vi "glb_static.vi"() -> ()   [LabVIEW 2014]
panel:
  in  "2-计算方法":string[](array[string])=["", "常数", "加", "减", "乘", "除", "微分", "积分", "幂运算", "散热量计算"]
  in  "2-变量来源_少运算":string[](array[string])=["", "测试模块1", "测试模块2", "测试模块3", "测试模块4", "测试模块5", "测试模块6", "测试模块7", "测试模块8", "cRIO", "GPS", "OBD", "冷却系统控制"]
  in  "2-变量来源_全部":string[](array[string])=["", "测试模块1", "测试模块2", "测试模块3", "测试模块4", "测试模块5", "测试模块6", "测试模块7", "测试模块8", "cRIO", "GPS", "OBD", "冷却系统控制", "运算"]
  in  "连接状态_OBD":bool
  in  "连接状态_GPS":bool
  in  "网络流2写入到的元素数量":i64
  in  "网络流2信息":T1={"cRIO名称"="RT", "读取方名称"="XpdGhnv3vatyoD3", "写入方名称 "="zGR2YhZf2vjoZ5U", "网络流大小"=10240, "网络流超时"=5000, "元素类型"={"消息"="", "数据"=variant}}
  in  "网络流2读取方端点":refnum<k21>
  in  "网络流1写入方端点":refnum<k21>
  in  "网络流1读取到的元素数量":i64
  in  "连接状态_cRIO":bool
  in  "连接状态_网络":bool
  out "测试模块储存文件引用":refnum<file>[](array[refnum])
  in  "数据储存—数据位置":string="data"
  in  "数据储存—试验信息目录":string="data\\testInfo.xls"
  in  "测试模块储存文件路径":path[](array[path])=[path "", path "", path "", path "", path "", path "", path "", path ""]
  in  "测试模块储存状态":bool[](array[boolean])=[FALSE, FALSE, FALSE, FALSE, FALSE, FALSE, FALSE, FALSE]
  in  "主界面配置":T2={"侧边栏数据"=[], "界面刷间隔率"=1000.0}
  in  "compactRIO配置":T3
  in  "GPS串口配置":T4={"串口资源名称"="", "波特率"=9600, "数据比特"=8, "奇偶"=0, "停止位"=15, "流控制"=0, "超时"=10000}
  in  "OBD串口配置":T4={"串口资源名称"="", "波特率"=9600, "数据比特"=8, "奇偶"=0, "停止位"=15, "流控制"=0, "超时"=10000}
  in  "用户信息":T5
  in  "所有URL":T6={"URL用户登录"="http://www.egreatcar.cn/Evehicle/user/checkUserLogin.php?account=value0&password=value1", "URL用户信息"="http://www.egreatcar.cn/Evehicle/user/getUserInfo.php?userID=value0", "URL历史数据创建数据表单"="http://www.egreatcar.cn/Evehicle/uploadHistory/createTestTable.php?query=value0", "URL历史数据上传试验信息"="http://www.egreatcar.cn/Evehicle/uploadHistory/uploadTestInfo.php?query=value0", "URL历史数据上传试验数据"="http://www.egreatcar.cn/Evehicle/uploadHistory/uploadTestData.php?query=value0", "URL实时数据上传"="http://www.egreatcar.cn/Evehicle/uploadRealtime/uploadRealtime.php?module1=value0&module2=value1&module3=value2&module4=value3&module5=value4&module6=value5&module7=value6&module8=value7", "URL=历史数据删除"="http://www.egreatcar.cn/Evehicle/uploadHistory/deleteOne.php", "URL=历史数据isExist"="http://www.egreatcar.cn/Evehicle/uploadHistory/checkExist.php", "URL=GPS位置"="http://www.egreatcar.cn/egreatcar/status/GPS.php?x=value0&y=value1"}
  in  "网络流1信息":T1={"cRIO名称"="RT", "读取方名称"="2ltITkYLm2nzMX4", "写入方名称 "="Ur9s1LsNrnvwwwr", "网络流大小"=10240, "网络流超时"=5000, "元素类型"={"消息"="", "数据"=variant}}
  in  "已打开模块":path[](array[path])
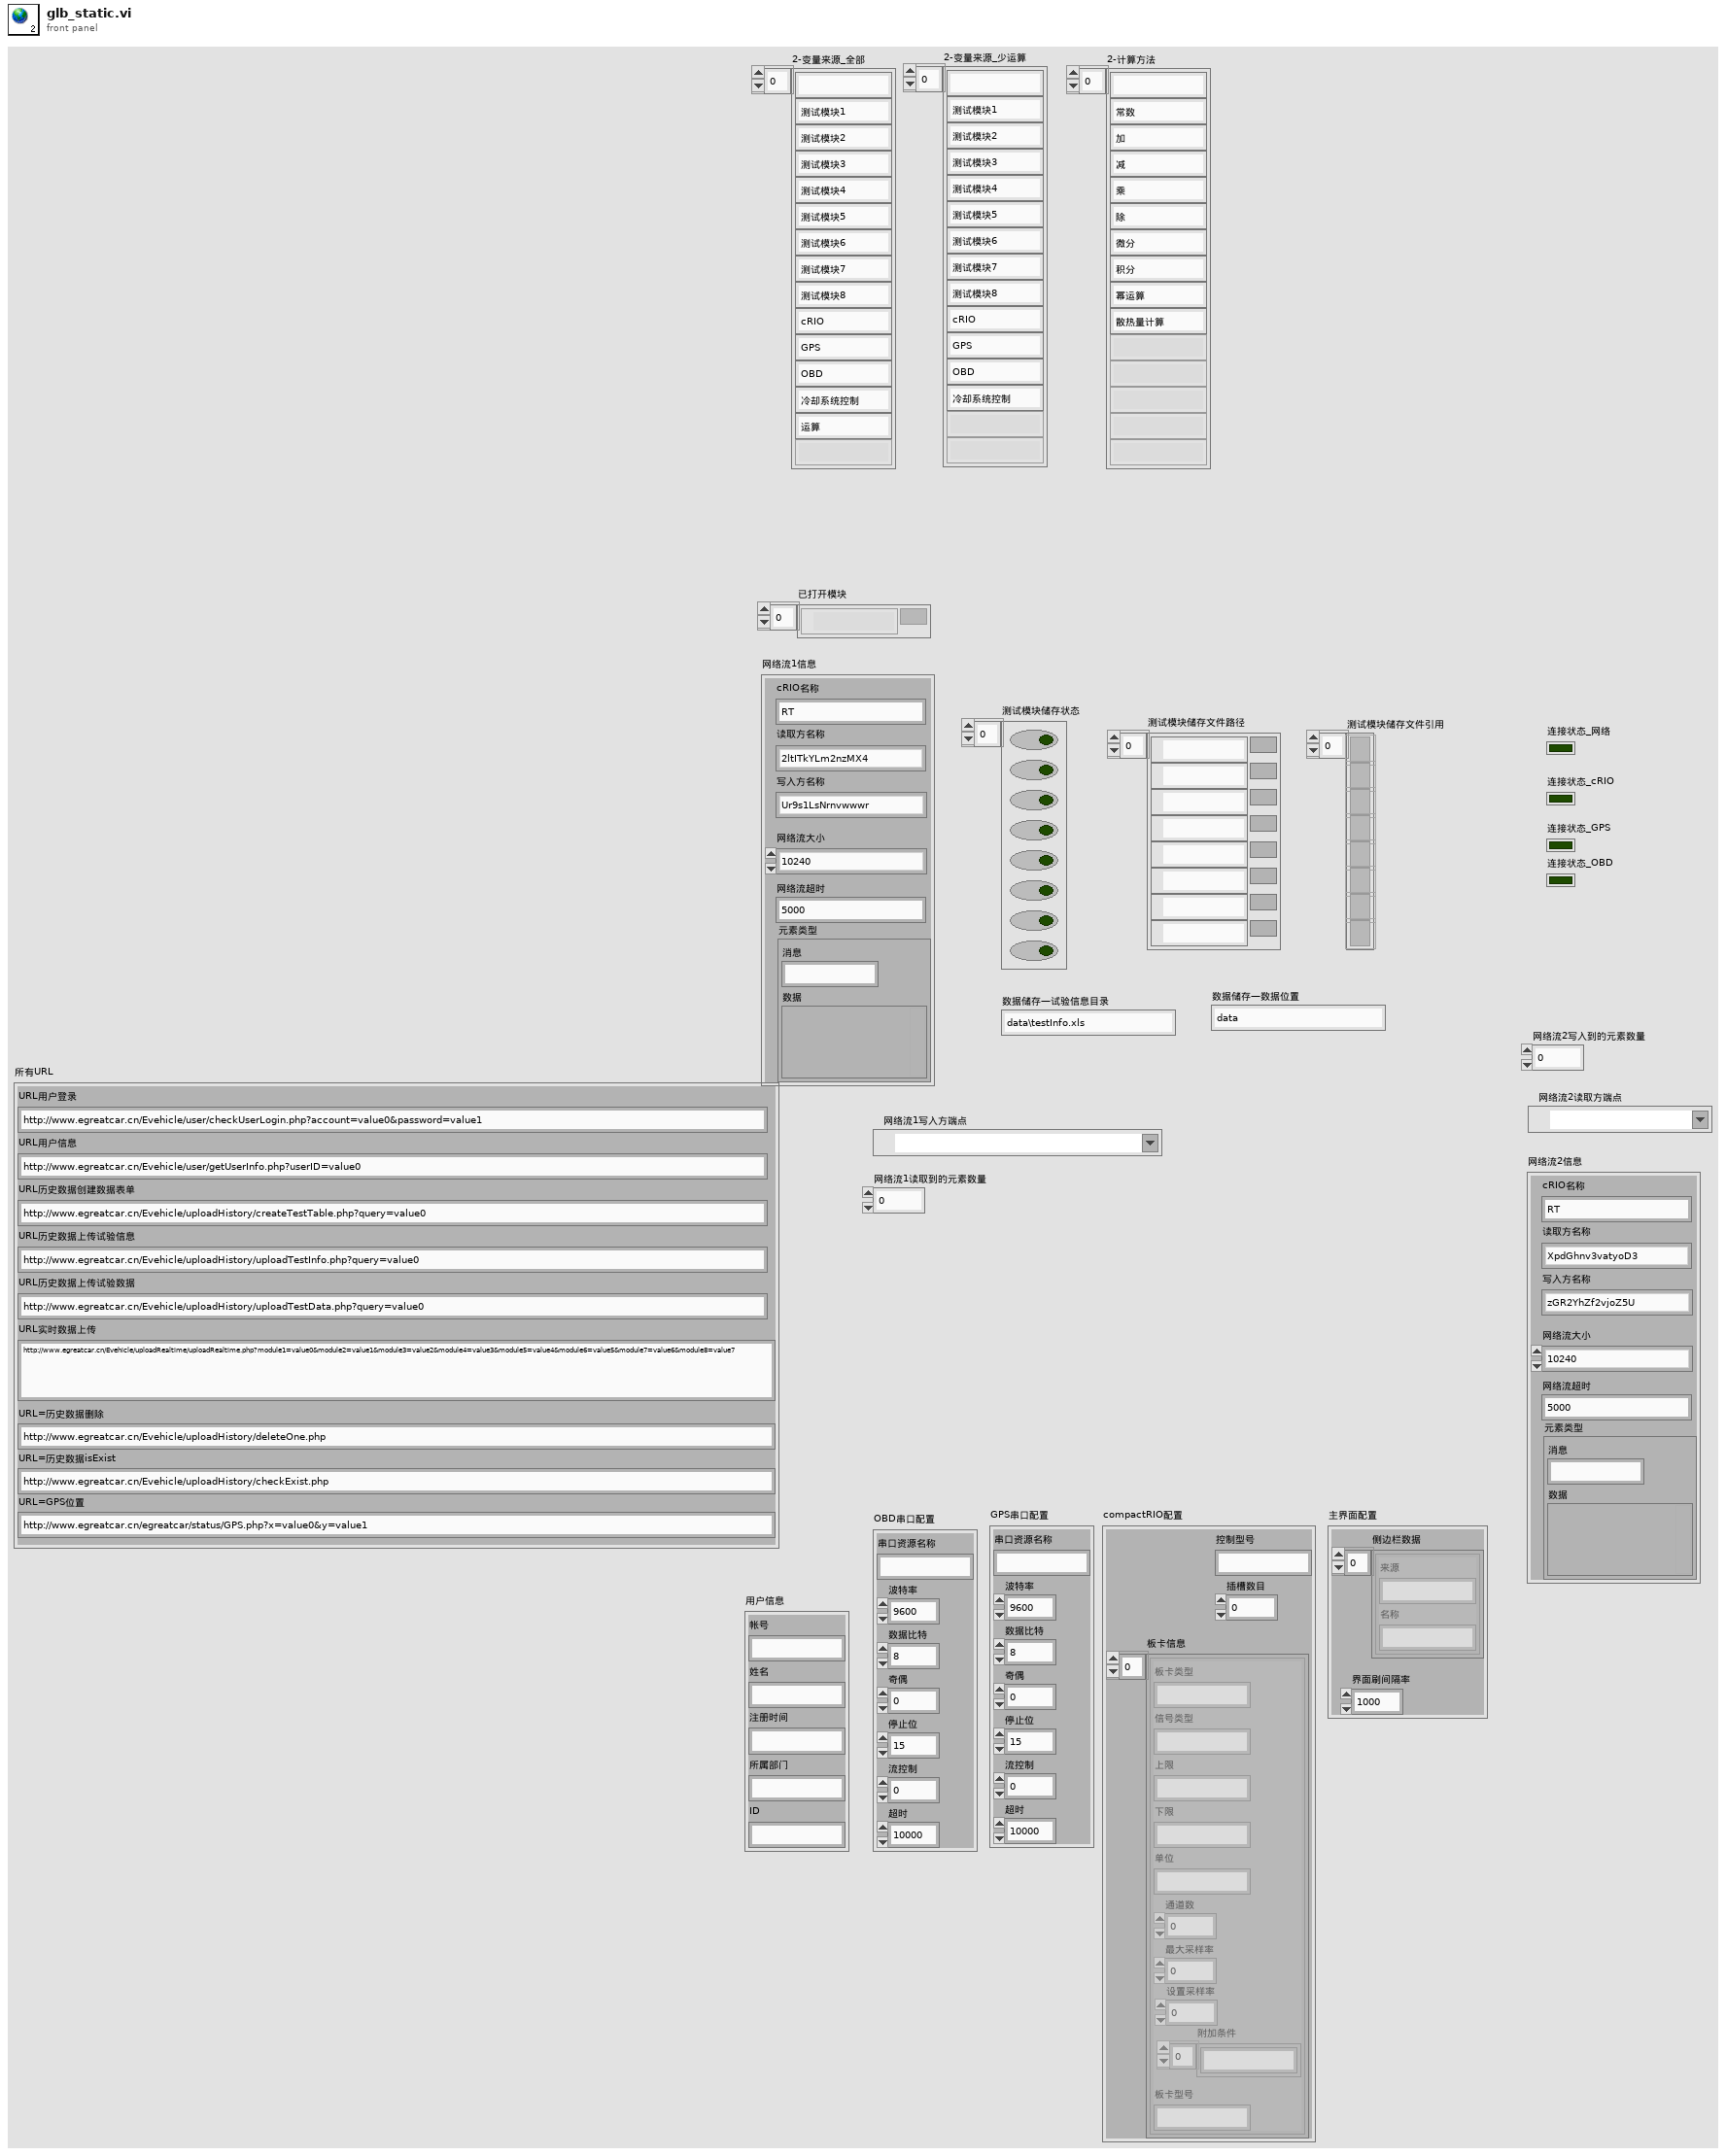
[diagram p1: front panel]
types:
  T1 = cluster{"cRIO名称":string, "读取方名称":string, "写入方名称 ":string, "网络流大小":i32, "网络流超时":i32, "元素类型":cluster{"消息":string, "数据":variant}}
  T2 = cluster{"侧边栏数据":cluster{"来源":string, "名称":string}[], "界面刷间隔率":dbl}
  T3 = cluster{"控制型号":string, "插槽数目":u32, "板卡信息":cluster{"板卡类型":string, "信号类型":string, "上限":string, "下限":string, "单位":string, "通道数":u32, "最大采样率":u32, "设置采样率":u32, "附加条件":string[], "板卡型号":string}[]}
  T4 = cluster{"串口资源名称":string, "波特率":u32, "数据比特":u32, "奇偶":u32, "停止位":u32, "流控制":u32, "超时":u32}
  T5 = cluster{"姓名":string, "注册时间":string, "所属部门":string, "ID":string, "帐号":string}
  T6 = cluster{"URL用户登录":string, "URL用户信息":string, "URL历史数据创建数据表单":string, "URL历史数据上传试验信息":string, "URL历史数据上传试验数据":string, "URL实时数据上传":string, "URL=历史数据删除":string, "URL=历史数据isExist":string, "URL=GPS位置":string}
diagram:
